vi "dot_product.vi"(10 "y":u32, 11 "x":u32) -> (3 "out":u64)   [LabVIEW 2017]
uses:
  <vilib>/rvi/FXPMathLib/SharedSubVIs/typedef/nifxpmath_BASIC_ImplementationSettings.ctl
  <vilib>/fxp/LVFixedPointQuantizationPolicyTypeDef.ctl
  <vilib>/fxp/LVFixedPointOverflowPolicyTypeDef.ctl
  <vilib>/rvi/ClientSDK/Core/DevComputerLib/Private/FourWireProtocol(cint64).vi
  <vilib>/rvi/FXPMathLib/FxpMultComplex/XNode/niFpgaMultComplex.xnode
  <vilib>/rvi/ClientSDK/Core/DevComputerLib/niFpgaDevCompUtilities.lvlib
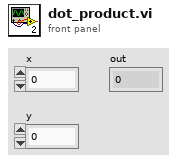
[diagram p1: front panel]
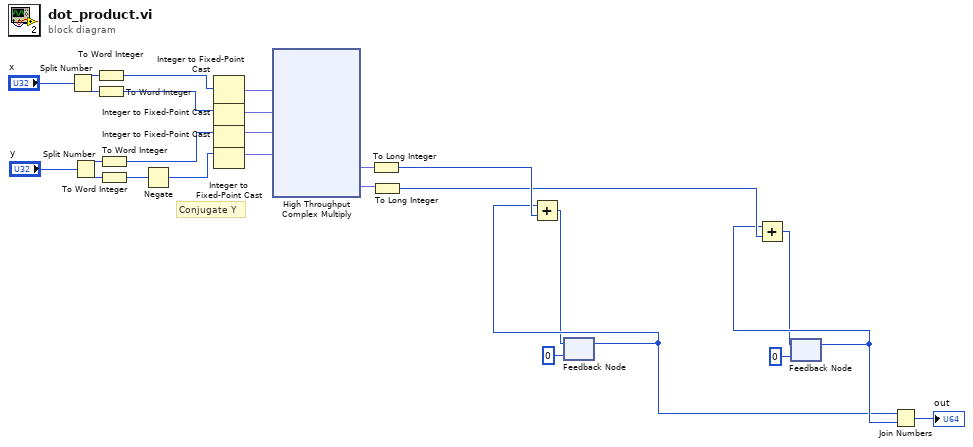
[diagram p0: block diagram]
diagram:
  # "Conjugate Y"
  n1 = Split Number(x="x") -> (hi(x)=w21:u16, lo(x)=w20:u16)
  n2 = Split Number(x="y") -> (hi(x)=w19:u16, lo(x)=w18:u16)
  n3 = To Word Integer(number=w21) -> (16bit integer=w14:i16)
  n4 = To Word Integer(number=w20) -> (16bit integer=w13:i16)
  n5 = To Word Integer(number=w19) -> (16bit integer=w12:i16)
  n6 = To Word Integer(number=w18) -> (16bit integer=w25:i16)
  n7 = Negate(x=w25) -> (-x=w26:i16)
  n8 = Integer to Fixed-Point Cast(integer=w14) -> (fixed-point=w15:fxp<+/-,16,16>)  [unwired: 1 in]
  n9 = Integer to Fixed-Point Cast(integer=w13) -> (fixed-point=w17:fxp<+/-,16,16>)  [unwired: 1 in]
  n10 = Integer to Fixed-Point Cast(integer=w12) -> (fixed-point=w16:fxp<+/-,16,16>)  [unwired: 1 in]
  n11 = Integer to Fixed-Point Cast(integer=w26) -> (fixed-point=w24:fxp<+/-,16,16>)  [unwired: 1 in]
  n12 = xnode "High Throughput Complex Multiply"("xr"=w15, "xi"=w17, "yr"=w16, "yi"=w24) -> ("pr"=w11:fxp<+/-,33,33>, "pi"=w10:fxp<+/-,33,33>)
  n13 = To Long Integer(number=w11) -> (32bit integer=w23:i32)
  n14 = To Long Integer(number=w10) -> (32bit integer=w22:i32)
  n15 = feedback #1(0) -> (w5:i32)
  n16 = Add(x=w5, y=w23) -> (x+y=w2:i32)
  n17 = feedback-in #1(w2) -> ()
  n18 = feedback #2(0) -> (w9:i32)
  n19 = Add(x=w9, y=w22) -> (x+y=w8:i32)
  n20 = feedback-in #2(w8) -> ()
  n21 = Join Numbers(hi=w5, lo=w9) -> ((hi.lo)=→"out":u64)
